vi "PPG_ABC.contents.vi"() -> ()   [LabVIEW 2014, in "PPG_ABC.lvlib"]
doc: "loads all VIs into memory - required for building an application"
uses:
  PPG_ABC.lvlib
panel:
  out "error out":errorcluster
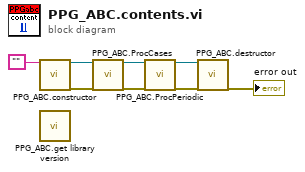
[diagram p0: block diagram]
diagram:
  n1 = call "PPG_ABC.constructor.vi"("name"="") -> ("i ref out"=w2:refnum<vi>, "error out"=w8:errorcluster)  [unwired: 16 in, 1 out]
  n2 = call "PPG_ABC.get library version.vi"() -> ()  [unwired: 1 in, 1 out]
  n3 = call "PPG_ABC.ProcCases.vi"("i ref in"=w2, "error in (no error)"=w8) -> ("i ref out"=w3:refnum<vi>, "error out"=w7:errorcluster)  [unwired: 15 in, 1 out]
  n4 = call "PPG_ABC.ProcPeriodic.vi"("i ref in"=w3, "error in (no error)"=w7) -> ("i ref out"=w4:refnum<vi>, "error out"=w6:errorcluster)  [unwired: 15 in, 1 out]
  n5 = call "PPG_ABC.destructor.vi"("i ref in"=w4, "error in(no error)"=w6) -> ("error out"=→"error out":errorcluster)  [unwired: 17 in]
